vi "ErrorCheckString.vi"(1 "Error String":string) -> (0 "Stop?":bool)   [LabVIEW 2014]
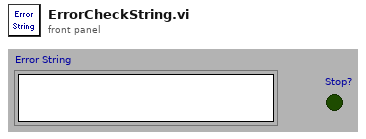
[diagram p1: front panel]
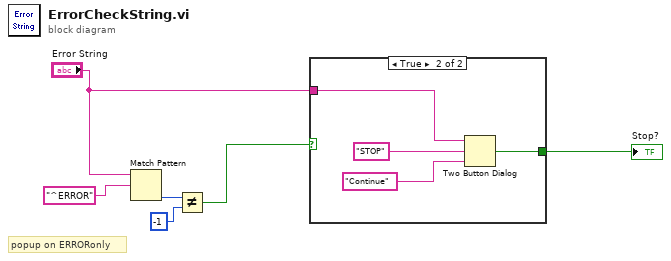
[diagram p0: block diagram]
diagram:
  # "popup on ERRORonly"
  n1 = Match Pattern(string="Error String", regular expression="^ERROR") -> (offset past match=w4:i32)  [unwired: 1 in, 3 out]
  n2 = Not Equal?(x=w4, y=-1) -> (x != y?=w2:bool)
  n3 = case shown="True" w2 {
    tunnel: "Error String" -> [_ w10]
    tunnel: [FALSE ("true") w9] -> w1
    frame False {
    }
    frame True {
      n4 = Two Button Dialog(message=w10, 1:"Continue" ("button name (\"OK\")"), 2:"STOP" ("T button name (\"OK\")")) -> (T button?=w9:bool)
    }
  }
  "Stop?" <- w1
